vi "ZMQ SUBSCRIBE (SubVI).vi"(8 "error in (no error)":errorcluster, 11 "output cluster":T1) -> (0 "error out":errorcluster)   [LabVIEW 2016]
uses:
  Que Cluster TD.ctl
  Que Atributes TD.ctl
  Que enum td.ctl
  Intrinsic data TD.ctl
  <vilib>/addons/zeromq/socket_type.ctl
  <vilib>/addons/zeromq/socket_options.ctl
  <vilib>/addons/zeromq/zeromq.lvlib
  <vilib>/addons/zeromq/zmq_context.lvclass
  <vilib>/addons/zeromq/zmq_socket.lvclass
panel:
  out "Intrinsic Data":cluster{dbl, dbl, dbl}(graph)
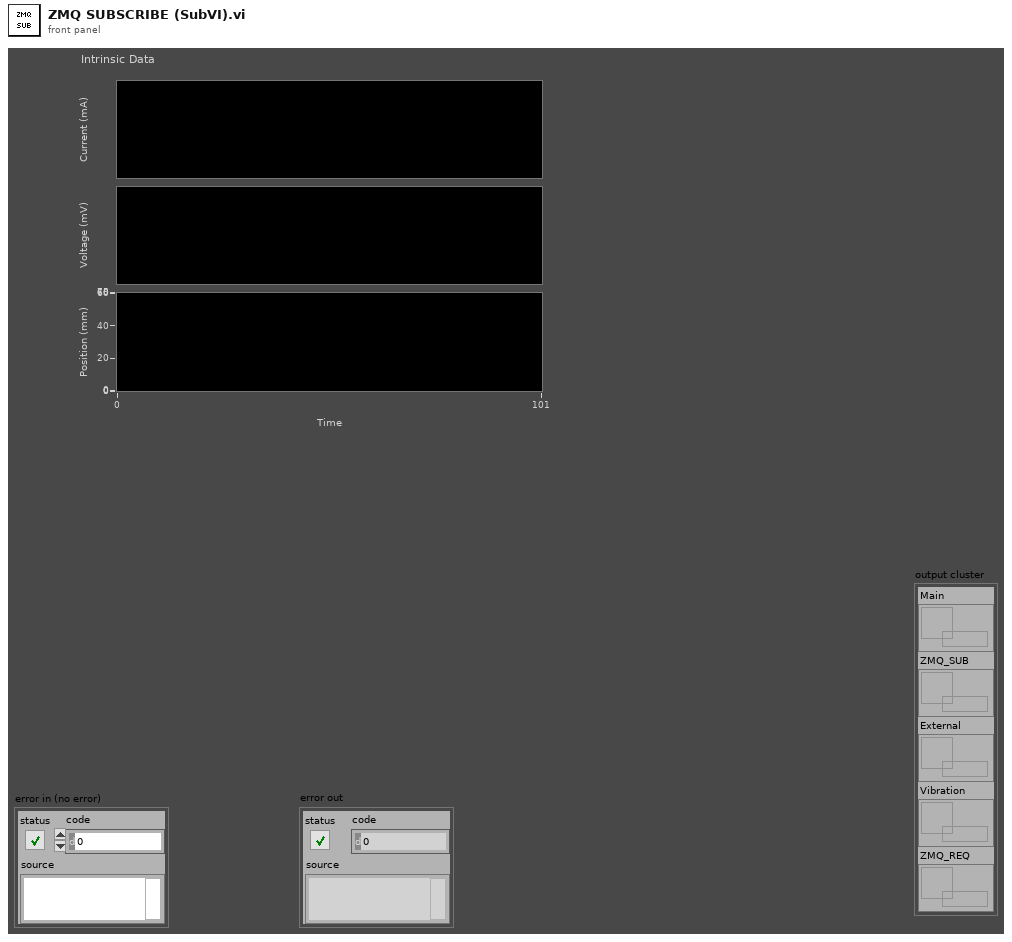
[diagram p1: front panel]
types:
  T1 = typedef "Que Cluster TD.ctl" = cluster{"Main":refnum<queue>, "ZMQ_SUB":refnum<queue>, "External":refnum<queue>, "Vibration":refnum<queue>, "ZMQ_REQ":refnum<queue>}
  T2 = typedef "Intrinsic data TD.ctl" = cluster{"Current TS":string, "Current Data":string, "Voltage TS":string, "Voltage Data":string, "Position TS":string, "Position Data":string, "Connected?":bool, "Log File Refnum":refnum<file>, "Logging?":bool, "Plot?":bool, "LV_C_TS":dbl, "LV_P_TS":dbl, "LV_V_TS":dbl}
  T3 = typedef "Que Atributes TD.ctl" = cluster{"Que States":T4, "String":string, "Boolean":bool, "Double":dbl, "U16":u16}
  T4 = typedef "Que enum td.ctl" = enum16{"Stop", "Start", "Update D_HW", "Initialize", "Exit", "Read", "Write", "Plot", "Log", "Stop Log", "Start Log", "Wait"}
  T5 = typedef "zeromq.lvlib/socket_options.ctl" = enum8{"NONE", "ZMQ_HWM", "<2>", "ZMQ_SWAP", "ZMQ_AFFINITY", "ZMQ_IDENTITY", "ZMQ_SUBSCRIBE", "ZMQ_UNSUBSCRIBE", "ZMQ_RATE", "ZMQ_RECOVERY_IVL", "ZMQ_MCAST_LOOP", "ZMQ_SNDBUF", "ZMQ_RCVBUF", "ZMQ_RCVMORE", "ZMQ_FD", "ZMQ_EVENTS", "ZMQ_TYPE", "ZMQ_LINGER", "ZMQ_RECONNECT_IVL", "ZMQ_BACKLOG", "ZMQ_RECOVERY_IVL_MSEC", "ZMQ_RECONNECT_IVL_MAX", "ZMQ_MAXMSGSIZE", "ZMQ_SNDHWM", "ZMQ_RCVHWM", "ZMQ_MULTICAST_HOPS", "<26>", "ZMQ_RCVTIMEO", "ZMQ_SNDTIMEO", "<29>", "<30>", "ZMQ_IPV4ONLY", "ZMQ_LAST_ENDPOINT", "ZMQ_ROUTER_MANDATORY", "ZMQ_TCP_KEEPALIVE", "ZMQ_TCP_KEEPALIVE_CNT", "ZMQ_TCP_KEEPALIVE_IDLE", "ZMQ_TCP_KEEPALIVE_INTVL", "ZMQ_TCP_ACCEPT_FILTER", "ZMQ_DELAY_ATTACH_ON_CONNECT", "ZMQ_XPUB_VERBOSE"}
  T6 = typedef "zeromq.lvlib/socket_type.ctl" = enum8{"ZMQ_PAIR", "ZMQ_PUB", "ZMQ_SUB", "ZMQ_REQ", "ZMQ_REP", "ZMQ_DEALER", "ZMQ_ROUTER", "ZMQ_PULL", "ZMQ_PUSH", "ZMQ_XPUB", "ZMQ_XSUB"}
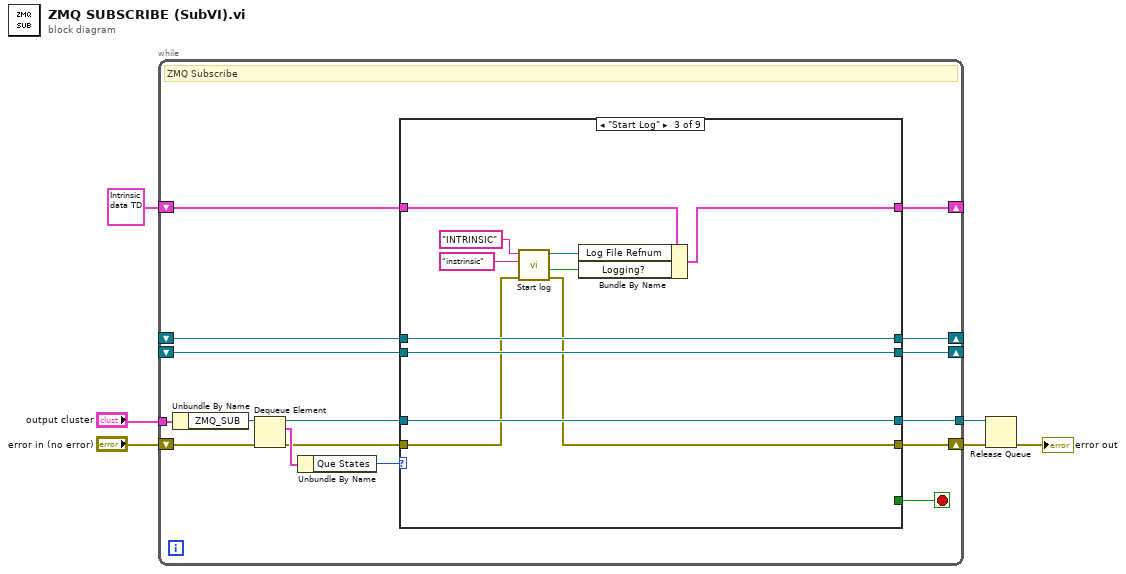
[diagram p0: block diagram]
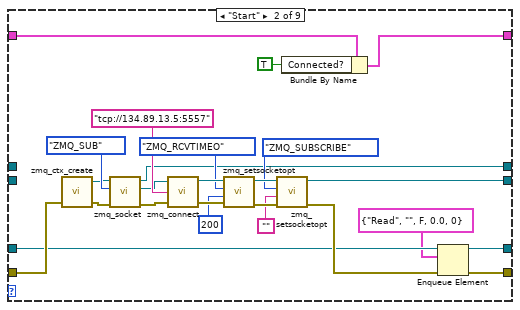
[diagram p3: hidden frame]
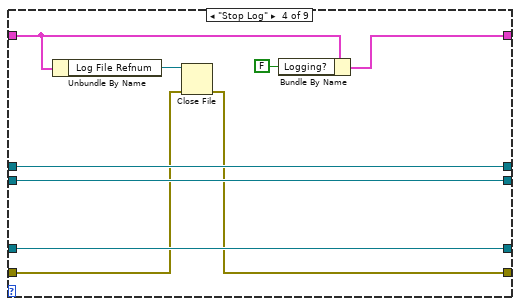
[diagram p4: hidden frame]
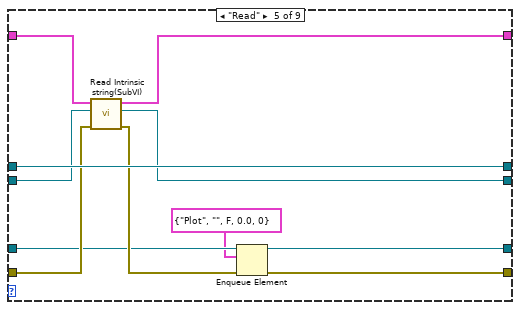
[diagram p5: hidden frame]
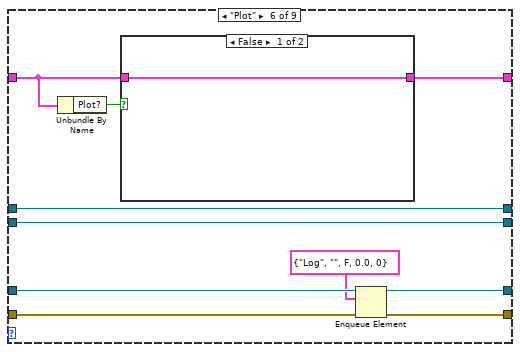
[diagram p6: hidden frame]
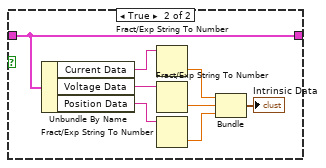
[diagram p7: hidden frame]
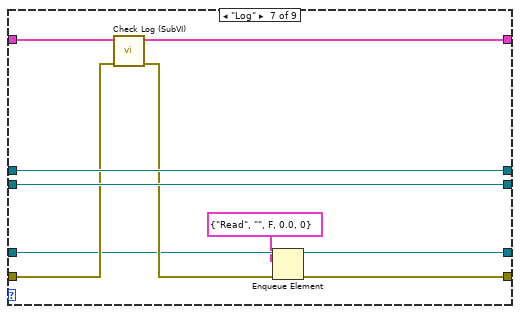
[diagram p8: hidden frame]
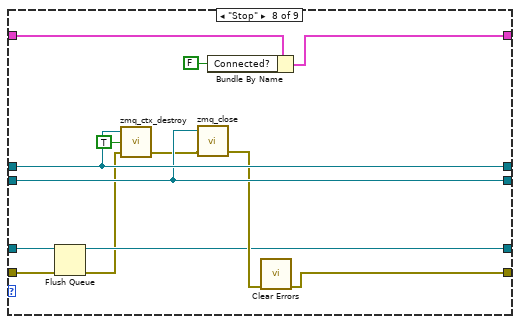
[diagram p9: hidden frame]
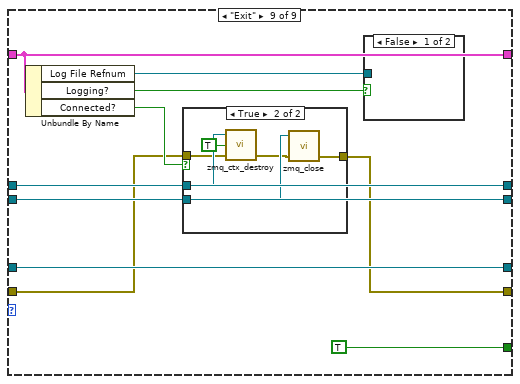
[diagram p10: hidden frame]
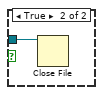
[diagram p11: hidden frame]
diagram:
  n1 = while {
    tunnel: "output cluster" -> [w22]
    tunnel: [w16] -> w5
    shift-right: [w15] -> w6
    shift-left: "error in (no error)" -> [w20]
    shift-right: [w12] -> _
    shift-left: _ -> [w11]
    shift-right: [w10] -> _
    shift-left: _ -> [w9]
    shift-right: [w7] -> _
    shift-left: T2 {"Current TS"="", "Current Data"="", "Voltage TS"="", "Voltage Data"="", "Position TS"="", "Position Data"="", "Connected?"=FALSE, "Log File Refnum"=refnum, "Logging?"=FALSE, "Plot?"=FALSE, "LV_C_TS"=0.0, "LV_P_TS"=0.0, "LV_V_TS"=0.0} ("Intrinsic Data Cluster TD") -> [w8]
    stop <- w13 stop-if-true
    # "ZMQ Subscribe"
    n2 = Unbundle By Name(w22) -> ("ZMQ_SUB"=w21:refnum<queue>)
    n3 = Dequeue Element(queue=w21, error in (no error)=w20) -> (queue out=w17:refnum<queue>, element=w19:T3, error out=w18:errorcluster)  [unwired: 1 in, 1 out]
    n4 = Unbundle By Name(w19) -> ("Que States"=w14:T4)
    n5 = case shown="\"Start Log\"" w14 {
      tunnel: w18 -> [w26 w52 w60 w69 w82 w91 w108 w117 w127]
      tunnel: w17 -> [w27 w35 w63 w72 w79 w89 w105 w119 w135]
      tunnel: [w27 w34 w63 w72 w78 w88 w104 w118 w135] -> w16
      tunnel: [w26 w36 w59 w68 w80 w90 w106 w121 w126] -> w15
      tunnel: [_ _ _ _ _ _ _ _ TRUE] -> w13
      tunnel: [w24 w32 w62 w71 w76 w93 w112 w124 w133] -> w12
      tunnel: w11 -> [w24 _ w62 w71 w77 w93 w112 w124 w133]
      tunnel: [w25 w31 w61 w70 w83 w92 w111 w125 w132] -> w10
      tunnel: w9 -> [w25 _ w61 w70 w83 w92 w111 w125 w132]
      tunnel: w8 -> [w23 w30 w56 w65 w75 w85 w110 w115 w129]
      tunnel: [w23 w29 w55 w64 w74 w86 w109 w114 w129] -> w7
      frame "Initialize", Default {
      }
      frame "Start" {
        n6 = call <vilib>:"zmq_ctx_create.vi"("error in"=w52) -> ("error out"=w44:errorcluster, "context out"=w43:refnum<class "zmq_context.lvclass">)  [unwired: 3 in]
        n7 = call <vilib>:"zmq_socket.vi"("error in"=w44, "socket type"=socket_type."ZMQ_SUB", "context in"=w43) -> ("error out"=w47:errorcluster, "socket out"=w46:refnum<class "zmq_socket.lvclass">, "context out"=w31:refnum<class "zmq_context.lvclass">)  [unwired: 2 in]
        n8 = call <vilib>:"zmq_connect.vi"("error in"=w47, "endpoint"="tcp://134.89.13.5:5557", "socket in"=w46) -> ("error out"=w51:errorcluster, "socket out"=w50:refnum<class "zmq_socket.lvclass">)  [unwired: 1 in]
        n9 = call <vilib>:"zmq_setsocketopt.vi"("error in"=w51, "value"=200, "option"=socket_options."ZMQ_RCVTIMEO", "socket in"=w50) -> ("error out"=w40:errorcluster, "socket out"=w41:refnum<class "zmq_socket.lvclass">)  [unwired: 2 in]
        n10 = call <vilib>:"zmq_setsocketopt.vi"("error in"=w40, "value"="", "option"=socket_options."ZMQ_SUBSCRIBE", "socket in"=w41) -> ("error out"=w37:errorcluster, "socket out"=w32:refnum<class "zmq_socket.lvclass">)  [unwired: 2 in]
        n11 = Bundle By Name(cluster=w30, "Connected?"=TRUE) -> (w29:T2)
        n12 = Enqueue Element(queue=w35, element=T3 {"Que States"=enum."Read", "String"="", "Boolean"=FALSE, "Double"=0.0, "U16"=0}, error in (no error)=w37) -> (queue out=w34:refnum<queue>, error out=w36:errorcluster)  [unwired: 1 in, 1 out]
      }
      frame "Start Log" {
        n13 = call "Start log.vi"("error in (no error)"=w60, "Data type"="instrinsic", "elative path"="INTRINSIC") -> ("error out"=w59:errorcluster, "Logging"=w53:bool, "Byte Stream File out"=w54:refnum<file>)  [unwired: 6 in]
        n14 = Bundle By Name(cluster=w56, "Log File Refnum"=w54, "Logging?"=w53) -> (w55:T2)
      }
      frame "Stop Log" {
        n15 = Unbundle By Name(w65) -> ("Log File Refnum"=w67:refnum<file>)
        n16 = Close File(refnum=w67, error in=w69) -> (error out=w68:errorcluster)  [unwired: 1 out]
        n17 = Bundle By Name(cluster=w65, "Logging?"=FALSE) -> (w64:T2)
      }
      frame "Read" {
        n18 = call "Read Intrinsic string(SubVI).vi"("error in (no error)"=w82, "zmq_socket in"=w77, "Intrinsic Data Cluster TD"=w75) -> ("error out"=w81:errorcluster, "zmq_socket out"=w76:refnum<class "zmq_socket.lvclass">, "Intrinsic Data Cluster TD 2"=w74:T2)  [unwired: 6 in]
        n19 = Enqueue Element(queue=w79, element=T3 {"Que States"=enum."Plot", "String"="", "Boolean"=FALSE, "Double"=0.0, "U16"=0}, error in (no error)=w81) -> (queue out=w78:refnum<queue>, error out=w80:errorcluster)  [unwired: 1 in, 1 out]
      }
      frame "Plot" {
        n20 = Unbundle By Name(w85) -> ("Plot?"=w84:bool)
        n21 = case shown="False" w84 {
          tunnel: w85 -> [w94 w95]
          tunnel: [w94 w95] -> w86
          frame False {
          }
          frame True {
            n22 = Unbundle By Name(w95) -> ("Current Data"=w102:string, "Voltage Data"=w101:string, "Position Data"=w100:string)
            n23 = Fract/Exp String To Number(string=w102) -> (number=w99:dbl)  [unwired: 3 in, 1 out]
            n24 = Fract/Exp String To Number(string=w101) -> (number=w98:dbl)  [unwired: 3 in, 1 out]
            n25 = Fract/Exp String To Number(string=w100) -> (number=w97:dbl)  [unwired: 3 in, 1 out]
            n26 = Bundle(w99, w98, w97) -> (→"Intrinsic Data":cluster{dbl, dbl, dbl})  [unwired: 1 in]
          }
        }
        n27 = Enqueue Element(queue=w89, element=T3 {"Que States"=enum."Log", "String"="", "Boolean"=FALSE, "Double"=0.0, "U16"=0}, error in (no error)=w91) -> (queue out=w88:refnum<queue>, error out=w90:errorcluster)  [unwired: 1 in, 1 out]
      }
      frame "Log" {
        n28 = call "Check Log (SubVI).vi"("error in (no error)"=w108, "Intrinsic Data Cluster TD in"=w110) -> ("error out"=w107:errorcluster, "Intrinsic Data Cluster TD out"=w109:T2)  [unwired: 8 in]
        n29 = Enqueue Element(queue=w105, element=T3 {"Que States"=enum."Read", "String"="", "Boolean"=FALSE, "Double"=0.0, "U16"=0}, error in (no error)=w107) -> (queue out=w104:refnum<queue>, error out=w106:errorcluster)  [unwired: 1 in, 1 out]
      }
      frame "Stop" {
        n30 = Flush Queue(queue=w119, error in (no error)=w117) -> (queue out=w118:refnum<queue>, error out=w116:errorcluster)  [unwired: 1 out]
        n31 = call <vilib>:"zmq_ctx_destroy.vi"("error in"=w116, "reap? (F)"=TRUE, "context in"=w125) -> ("error out"=w123:errorcluster)  [unwired: 2 in]
        n32 = call <vilib>:"zmq_close.vi"("error in"=w123, "socket"=w124) -> ("error out"=w122:errorcluster)  [unwired: 3 in]
        n33 = Bundle By Name(cluster=w115, "Connected?"=FALSE) -> (w114:T2)
        n34 = call <vilib>:"Clear Errors.vi"("error in (no error)"=w122) -> ("error out"=w121:errorcluster)  [unwired: 5 in, 1 out]
      }
      frame "Exit" {
        n35 = Unbundle By Name(w129) -> ("Log File Refnum"=w128:refnum<file>, "Logging?"=w130:bool, "Connected?"=w131:bool)
        n36 = case shown="True" w131 {
          tunnel: w133 -> [_ w143]
          tunnel: w132 -> [_ w142]
          tunnel: w127 -> [w137 w141]
          tunnel: [w137 w139] -> w126
          frame False {
          }
          frame True {
            n37 = call <vilib>:"zmq_ctx_destroy.vi"("error in"=w141, "reap? (F)"=TRUE, "context in"=w142) -> ("error out"=w140:errorcluster)  [unwired: 2 in]
            n38 = call <vilib>:"zmq_close.vi"("error in"=w140, "socket"=w143) -> ("error out"=w139:errorcluster)  [unwired: 3 in]
          }
        }
        n39 = case shown="False" w130 {
          tunnel: w128 -> [_ w136]
          frame False {
          }
          frame True {
            n40 = Close File(refnum=w136) -> ()  [unwired: 1 in, 2 out]
          }
        }
      }
    }
  }
  n41 = Release Queue(queue=w5, error in (no error)=w6) -> (error out=→"error out":errorcluster)  [unwired: 1 in, 2 out]
